vi "ClosePort.vi"(0 "handle":i32) -> ()   [LabVIEW 2014, in "Sixpack - Driver.lvlib"]
uses:
  Sixpack - Driver.lvlib
  DLL/PackDLL.dll
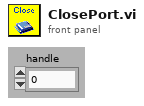
[diagram p1: front panel]
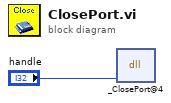
[diagram p0: block diagram]
diagram:
  n1 = dll-call lib="D:/CS-Source/LV2014/GPL/instr.lib/SixPack/PackDLL/DLL/PackDLL.dll" fn="_ClosePort@4" label="ClosePort"("HANDLE"="handle") -> ()  [unwired: 5 in, 2 out]
